vi "AnalogIO.vi"() -> ()   [LabVIEW 2011]
uses:
  <vilib>/Platform/TimedLoop/XDataNode/timing_clust.ctl
  <vilib>/Platform/TimedLoop/XDataNode/nitl_modes.ctl
  <vilib>/Platform/TimedLoop/XDataNode/wakeup.ctl
  <vilib>/Utility/error.llb/DialogType.ctl
  <vilib>/DAQmx/read.llb/DAQmx Read (Analog 2D DBL NChan NSamp).vi
  <vilib>/DAQmx/write.llb/DAQmx Write (Analog 1D DBL NChan 1Samp).vi
  <vilib>/DAQmx/create/channels.llb/DAQmx Create Channel (AI-Voltage-Basic).vi
  <vilib>/DAQmx/configure/timing.llb/DAQmx Timing (Sample Clock).vi
  <vilib>/Utility/file.llb/Write To Spreadsheet File (DBL).vi
  <vilib>/DAQmx/miscellaneous.llb/DAQmx Fill In Error Info.vi
  <vilib>/Platform/TimedLoop/XDataNode/XDataNode.xnode
  <vilib>/Platform/TimedLoop/XDataNode/XDNodeRunTimeDep.lvlib
panel:
  out "Time":dbl
  in  "Frequency 3":dbl=1.0
  in  "Amplitude 3":dbl[](array[numeric])=[1.8, 0.0, 0.0]
  out "Piezo driver input":T1(graph)
  out "Capacitive Sensor":T2(graph)
  in  "stop":bool
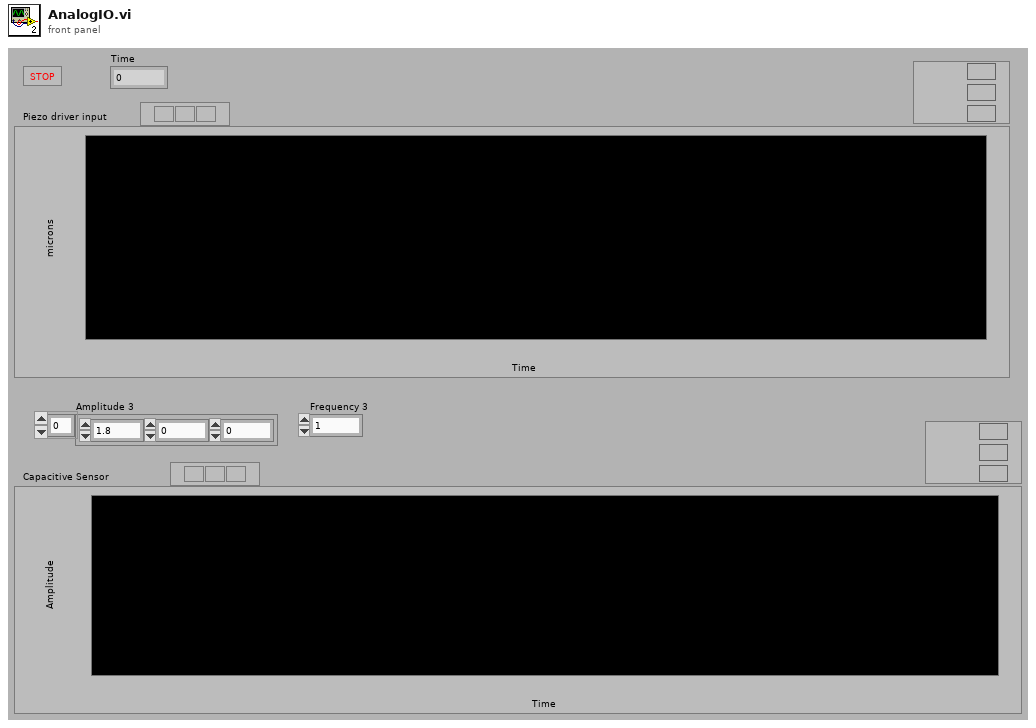
[diagram p1: front panel]
types:
  T1 = cluster{"dataOut[0]":dbl, "dataOut[1]":dbl, "dataOut[2]":dbl, "dataOut[3]":dbl, "dataOut[4]":dbl, "dataOut[5]":dbl, "dataOut[6]":dbl, "dataOut[7]":dbl, "dataOut[8]":dbl}
  T2 = cluster{"[0]":dbl, "[1]":dbl, "[2]":dbl, "[3]":dbl, "[4]":dbl, "[5]":dbl, "[6]":dbl, "[7]":dbl, "[8]":dbl}
  T3 = typedef "DialogType.ctl" = u16
  T4 = typedef "XDNodeRunTimeDep.lvlib/timing_clust.ctl" = cluster{"Expected End [f-1]":u64, "Actual End [f-1]":u64, "Finished Late? [f-1]":bool, "Expected End [i-1]":u64, "Actual End [i-1]":u64, "Finished Late? [i-1]":bool, "Expected Start [i]":u64, "Actual Start [i]":u64, "Expected Start [f]":u64, "Actual Start [f]":u64, "Source Name":string, "Structure Name":string, "Period":i64, "Deadline":i64, "Offset":i64, "Start":i64, "Priority":i32, "Timeout":i32, "Mode":T5, "Wakeup Reason":T6, "Error":errorcluster, "Source Type":string, "Secondary Source Type":string, "Global End Time":u64, "Global Start Time":u64, "Frame Duration":u64, "Iteration Duration":u64, "Assigned CPU":i32, "I/O Scan Engine Mode":u32}
  T5 = typedef "XDNodeRunTimeDep.lvlib/nitl_modes.ctl" = enum32{"No Change", "Process missed periods, maintain original phase", "Discard missed periods, maintain original phase", "Process missed periods, ignore original phase", "Discard missed periods, ignore original phase"}
  T6 = typedef "XDNodeRunTimeDep.lvlib/wakeup.ctl" = enum32{"Normal", "Aborted", "Asynchronous wakeup", "Timing source error", "Timed loop error", "Timeout"}
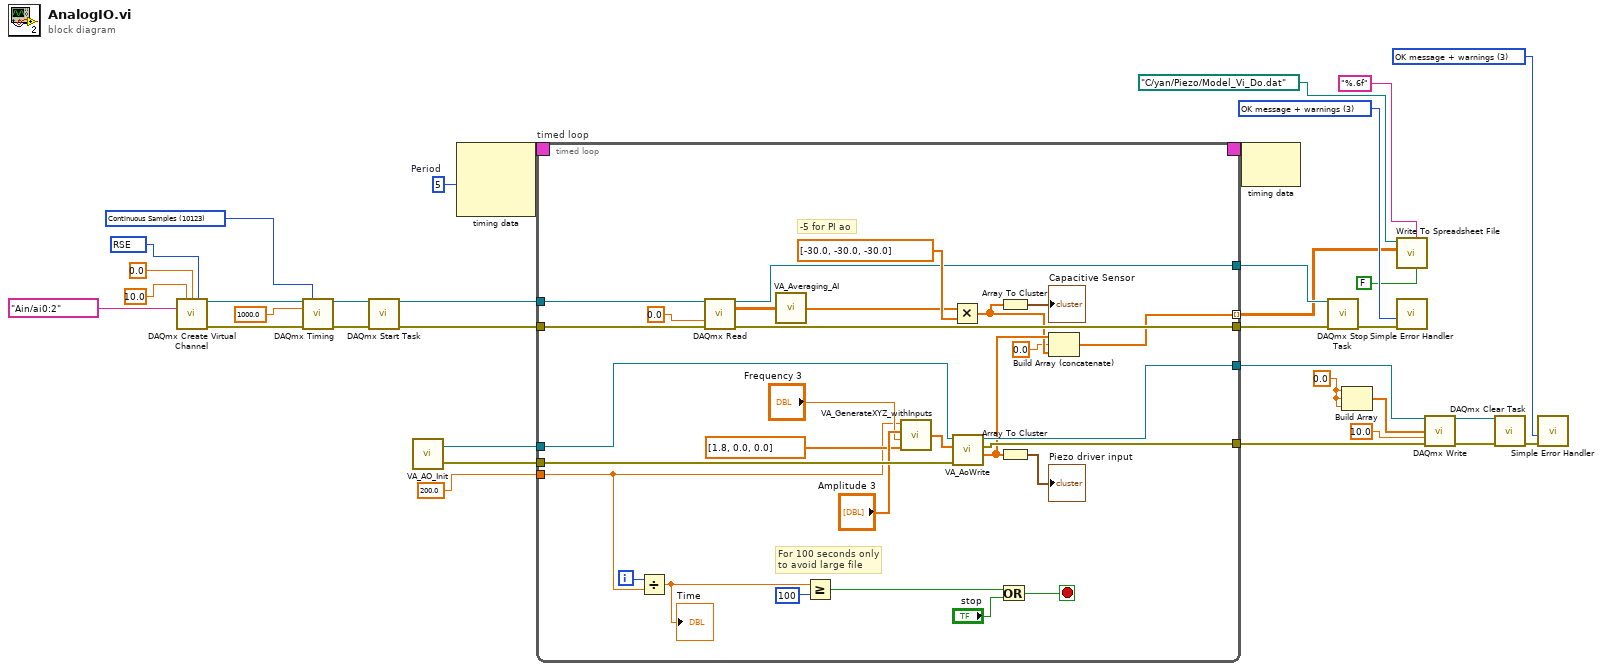
[diagram p0: block diagram]
diagram:
  w10 = 0.0 ("element")
  w13 = T3 3 items=["no dialog", "OK message", "continue or stop message", "OK message + warnings", "continue/stop + warnings"] ("type of dialog (OK msg:1)")
  w20 = T3 3 items=["no dialog", "OK message", "continue or stop message", "OK message + warnings", "continue/stop + warnings"] ("type of dialog (OK msg:1)")
  w27 = 10123 items=["Finite Samples"=10178, "Continuous Samples"=10123, "Hardware Timed Single Point"=12522] ("sample mode")
  w32 = 10083 items=["default"=-1, "RSE"=10083, "NRSE"=10078, "Differential"=10106, "Pseudodifferential"=12529] ("input terminal configuration")
  w33 = i64 5  # Period
  n1 = call-poly <vilib>:"DAQmx Create Virtual Channel.vi"("maximum value"=10.0, "minimum value"=0.0, "input terminal configuration"=w32, "physical channels"=tag "Ain/ai0:2") -> ("task out"=w29:refnum<k21>, "error out"=w28:errorcluster)  [unwired: 10 in]
  n2 = call-poly <vilib>:"DAQmx Timing.vi"("task/channels in"=w29, "sample mode"=w27, "rate"=1000.0, "error in"=w28) -> ("task out"=w25:refnum<k21>, "error out"=w24:errorcluster)  [unwired: 10 in]
  n3 = call <vilib>:"DAQmx Start Task.vi"("task/channels in"=w25, "error in"=w24) -> ("task out"=w22:refnum<k21>, "error out"=w21:errorcluster)  [unwired: 12 in]
  n4 = call "VA_AO_Init.vi"() -> ("error out"=w6:errorcluster, "task out"=w7:refnum<k21>)
  n5 = node-c288(w33) -> (w35:T4)  [unwired: 2 out]
  n6 = timed-loop "timed loop" {
    timing: w35 -> [_]
    timing-out: [_] -> w34
    tunnel: w22 -> [w60]
    tunnel: w21 -> [w59]
    tunnel: [w58] -> w18
    tunnel: [w57] -> w17
    tunnel: [w53] -> w9
    tunnel: [w52] -> w8
    tunnel: w7 -> [w55]
    tunnel: w6 -> [w54]
    tunnel: 200.0 ("SampleFrequency") -> [w38]
    tunnel: [w42] -> w1 mode=indexing
    i -> [w39]
    stop <- w37 stop-if-true
    # "For 100 seconds only\nto avoid large file"
    # "-5 for PI ao"
    n7 = Divide(x=w39, y=w38) -> (x/y=w40:dbl)
    "Time" <- w40
    n8 = call-poly <vilib>:"DAQmx Read.vi"("task/channels in"=w60, "timeout"=0.0, "error in"=w59) -> ("task out"=w57:refnum<k21>, "data"=w47:dbl[][], "error out"=w58:errorcluster)  [unwired: 10 in]
    n9 = call "VA_Averaging_AI.vi"("AnalogIn"=w47) -> ("Anolog XYZ"=w46:dbl[])
    n10 = Greater Or Equal?(x=w40, y=100) -> (x >= y?=w36:bool)
    n11 = call "VA_GenerateXYZ_withInputs.vi"("Bias"=dbl[] [1.8, 0.0, 0.0] ("Amplitude"), "Frequency"="Frequency 3", "Amplitude"="Amplitude 3", "SampleFrequency"=w38) -> ("xyz"=w48:dbl[])
    n12 = Multiply(x=w46, y=dbl[] [-30.0, -30.0, -30.0]) -> (x*y=w44:dbl[])
    n13 = call "VA_AoWrite.vi"("error in"=w54, "data"=w48, "task/channels in"=w55) -> ("dataOut"=w45:dbl[], "error out"=w52:errorcluster, "task out"=w53:refnum<k21>)  [unwired: 2 in]
    n14 = Or(x=w36, y="stop") -> (x .or. y?=w37:bool)
    n15 = Array To Cluster(array=w44) -> (cluster=→"Capacitive Sensor":T2)
    n16 = Array To Cluster(array=w45) -> (cluster=→"Piezo driver input":T1)
    n17 = Build Array (concatenate)(w45, 0.0 ("timeout"), w44) -> (w42:dbl[])
  }
  n18 = node-c288(w34) -> ()  [unwired: 1 out]
  n19 = call <vilib>:"DAQmx Stop Task.vi"("task/channels in"=w17, "error in"=w18) -> ("error out"=w19:errorcluster)  [unwired: 12 in, 1 out]
  n20 = Build Array(w10, w10, w10) -> (w11:dbl[])
  n21 = call-poly <vilib>:"Write To Spreadsheet File.vi"("transpose? (no:F)"=FALSE, "format (%.3f)"="%.6f" ("format (%d)"), "2D data"=w1, "file path (dialog if empty)"=path "C:/yan/Piezo/Model_Vi_Do.dat") -> ()  [unwired: 4 in, 1 out]
  n22 = call <vilib>:"Simple Error Handler.vi"("type of dialog (OK msg:1)"=w20, "error in (no error)"=w19) -> ()  [unwired: 3 in, 5 out]
  n23 = call-poly <vilib>:"DAQmx Write.vi"("task/channels in"=w9, "data"=w11, "timeout"=10.0, "error in"=w8) -> ("task out"=w15:refnum<k21>, "error out"=w14:errorcluster)  [unwired: 9 in, 1 out]
  n24 = call <vilib>:"DAQmx Clear Task.vi"("task in"=w15, "error in"=w14) -> ("error out"=w12:errorcluster)  [unwired: 13 in]
  n25 = call <vilib>:"Simple Error Handler.vi"("type of dialog (OK msg:1)"=w13, "error in (no error)"=w12) -> ()  [unwired: 3 in, 5 out]
